vi "Timer_gettime.vi"(8 "error in (no error)":errorcluster caption="错误输入（无错误）", 11 "Timer 输入":refnum<class "Timer.lvclass">) -> (0 "error out":errorcluster caption="错误输出", 2 "time":cluster{"计时？":bool, "计时 (ms)":u32}, 3 "Timer 输出":refnum<class "Timer.lvclass">)   [LabVIEW 2019, in "Timer.lvclass"]
uses:
  Timer.lvclass
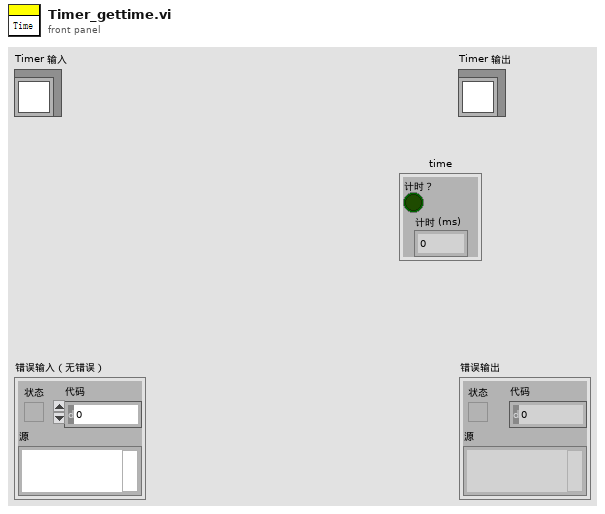
[diagram p1: front panel]
types:
  T1 = typedef "Timer.lvclass/Attribute.ctl" = cluster{"计时？":bool, "计时 (ms)":u32, "停止通知":refnum<notifier>}
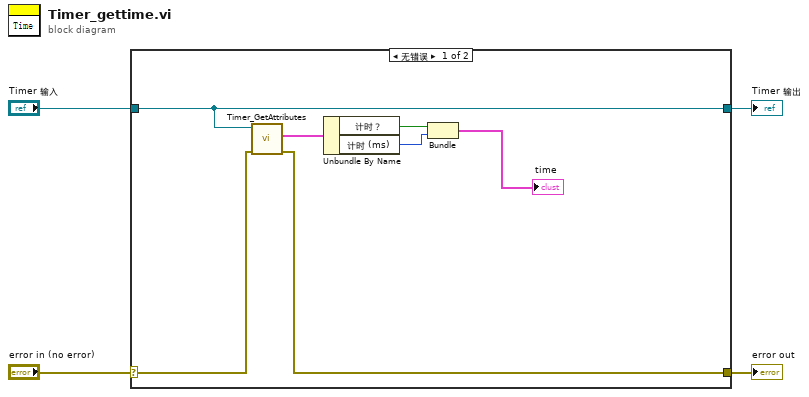
[diagram p0: block diagram]
diagram:
  n1 = case shown="无错误" "error in (no error)" {
    selector: "error in (no error)" -> [w6 w13]
    tunnel: [w5 w13] -> w3
    tunnel: [w11 w12] -> w1
    tunnel: "Timer 输入" -> [w11 w12]
    frame No Error {
      n2 = call "Timer_GetAttributes.vi"("error in (no error)"=w6, "Timer 输入"=w11) -> ("error out"=w5:errorcluster, "attribute"=w10:T1)  [unwired: 6 in, 2 out]
      n3 = Unbundle By Name(w10) -> ("计时？"=w9:bool, "计时 (ms)"=w8:u32)
      n4 = Bundle("计时？"=w9, "计时 (ms)"=w8) -> (→"time":cluster{"计时？":bool, "计时 (ms)":u32})  [unwired: 1 in]
    }
    frame Error {
    }
  }
  "error out" <- w3
  "Timer 输出" <- w1
